vi "Power_Supply Get Reference.vi"(8 "error in (no error)":errorcluster, 11 "Instrument Reference":u8) -> (0 "error out":errorcluster, 2 "Class Attributes":T1, 3 "Power_Supply Virtual.lvclass":refnum<class "Power_Supply Virtual.lvclass">)   [LabVIEW 2018, in "Power_Supply Virtual.lvclass"]
uses:
  Power_Supply Virtual.lvclass
  Controls/Class Attributes Cluster.ctl
  Power_Supply Global.vi
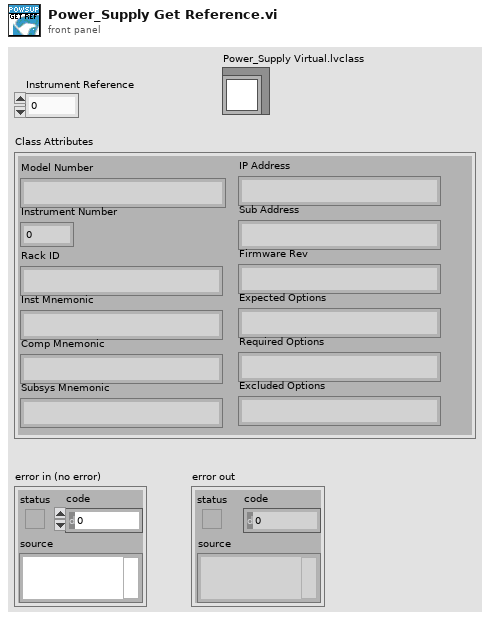
[diagram p1: front panel]
types:
  T1 = typedef "Class Attributes Cluster.ctl" = cluster{"Model Number":string, "Instrument Number":u8, "Rack ID":string, "Inst Mnemonic":string, "Comp Mnemonic":string, "Subsys Mnemonic":string, "IP Address":string, "Sub Address":string, "Firmware Rev":string, "Expected Options":string, "Required Options":string, "Excluded Options":string}
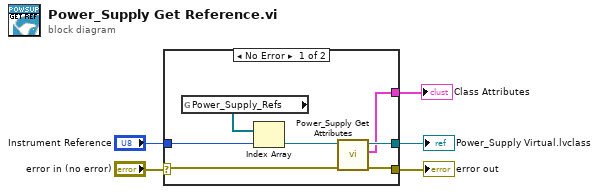
[diagram p0: block diagram]
diagram:
  n1 = case shown="No Error" "error in (no error)" {
    selector: "error in (no error)" -> [w9 w13]
    tunnel: [w10 w13] -> w4
    tunnel: "Instrument Reference" -> [w11 _]
    tunnel: [w7 _] -> w2
    tunnel: [w6 _] -> w1
    frame No Error {
      n2 = global read "Power_Supply Global.vi" "Power_Supply_Refs"() -> (w12:refnum<class "Power_Supply Virtual.lvclass">[])
      n3 = Index Array(array=w12, index=w11) -> (element=w8:refnum<class "Power_Supply Virtual.lvclass">)
      n4 = call-dynamic "Power_Supply Get Attributes.vi"("error in (no error)"=w9, "Power_Supply Virtual in"=w8) -> ("error out"=w10:errorcluster, "Class Attributes"=w6:T1, "Power_Supply Virtual out"=w7:refnum<class "Power_Supply Virtual.lvclass">)  [unwired: 7 in]
    }
    frame Error {
    }
  }
  "error out" <- w4
  "Power_Supply Virtual.lvclass" <- w2
  "Class Attributes" <- w1
